vi "ma_scale multitone amplitude.vi"(2 "amplitude":dbl, 3 "scaling method":enum16{"max absolute value", "peak detect"}(ring)=enum."peak detect", 4 "multitone in":dbl[](array[numeric])) -> (0 "crest factor":dbl, 1 "multitoneout":dbl[](array[numeric]))   [LabVIEW 2020, in "NI_MAPro.lvlib"]
uses:
  NI_MAPro.lvlib
  NI_AALPro.lvlib
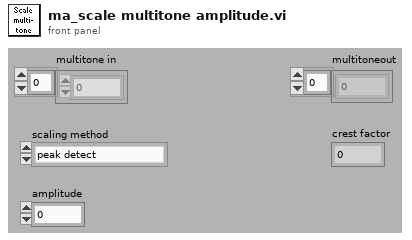
[diagram p1: front panel]
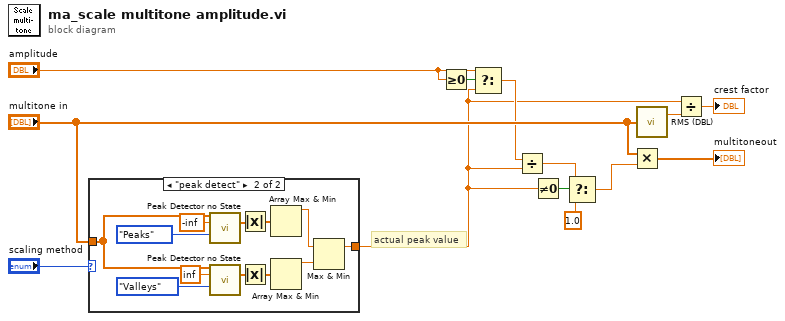
[diagram p0: block diagram]
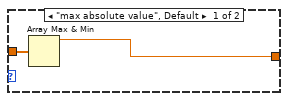
[diagram p2: hidden frame]
diagram:
  # "actual peak value"
  n1 = case shown="\"peak detect\"" "scaling method" {
    tunnel: [w14 w16] -> w5
    tunnel: "multitone in" -> [w15 w17]
    frame "max absolute value", Default {
      n2 = Array Max & Min(array=w15) -> (max value=w14:dbl)  [unwired: 3 out]
    }
    frame "peak detect" {
      n3 = call "Peak Detector no State.vi"("X"=w17, "threshold"=-inf, "peaks/valleys"=enum32{"Peaks", "Valleys"}."Peaks") -> ("Amplitudes"=w22:dbl[])  [unwired: 5 in, 7 out]
      n4 = call "Peak Detector no State.vi"("X"=w17, "threshold"=inf, "peaks/valleys"=enum32{"Peaks", "Valleys"}."Valleys") -> ("Amplitudes"=w23:dbl[])  [unwired: 5 in, 7 out]
      n5 = Absolute Value(x=w22) -> (abs(x)=w20:dbl[])
      n6 = Absolute Value(x=w23) -> (abs(x)=w21:dbl[])
      n7 = Array Max & Min(array=w20) -> (max value=w19:dbl)  [unwired: 3 out]
      n8 = Array Max & Min(array=w21) -> (max value=w18:dbl)  [unwired: 3 out]
      n9 = Max & Min(x=w19, y=w18) -> (max(x,y)=w16:dbl)  [unwired: 1 out]
    }
  }
  n10 = Greater Or Equal To 0?(x="amplitude") -> (x >= 0?=w8:bool)
  n11 = Select(t="amplitude", s=w8, f=w5) -> (s? t:f=w6:dbl)
  n12 = Divide(x=w6, y=w5) -> (x/y=w2:dbl)
  n13 = Not Equal To 0?(x=w5) -> (x != 0?=w4:bool)
  n14 = Select(t=w2, s=w4, f=1.0) -> (s? t:f=w1:dbl)
  n15 = Multiply(x="multitone in", y=w1) -> (x*y=→"multitoneout":dbl[])
  n16 = call "RMS (DBL).vi"("X"="multitone in") -> ("rms value"=w11:dbl)  [unwired: 1 out]
  n17 = Divide(x=w5, y=w11) -> (x/y=→"crest factor":dbl)
